vi "Get column name.vi"(8 "error in (no error)":errorcluster, 11 "Column in":refnum<class "Column.lvclass">) -> (0 "error out":errorcluster, 2 "Column Name":string, 3 "Column out":refnum<class "Column.lvclass">)   [LabVIEW 2020, in "Basic Columns.lvlib" / "Column.lvclass"]
uses:
  Column.lvclass
  Column.lvclass/Column.ctl
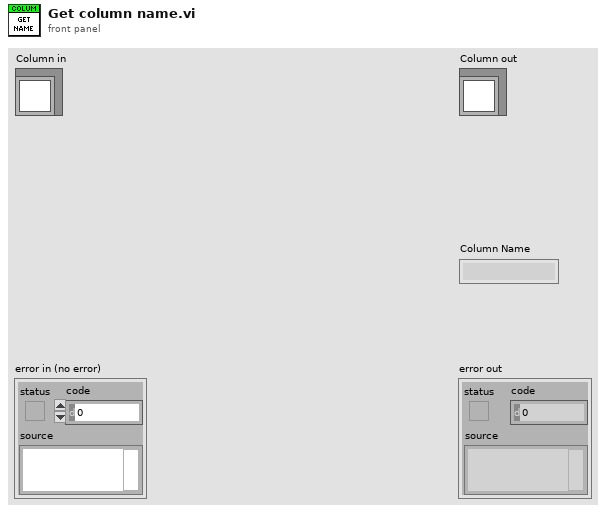
[diagram p1: front panel]
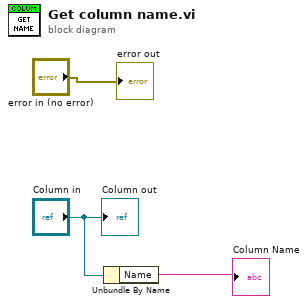
[diagram p0: block diagram]
diagram:
  n1 = Unbundle By Name("Column in") -> ("Name"=→"Column Name":string)
  "error out" <- "error in (no error)"
  "Column out" <- "Column in"
